vi "Motor_ReadPIDGains.vi"(8 "error in (no error)":errorcluster, 11 "MotorNew in":refnum<class "MotorControl.lvclass">) -> (0 "error out":errorcluster, 2 "PID Gains":T1(array[cluster]), 3 "MotorNew out":refnum<class "MotorControl.lvclass">)   [LabVIEW 2014, in "MotorControl.lvclass"]
uses:
  MotorControl.lvclass
  MotorControl.lvclass/MotorControl.ctl
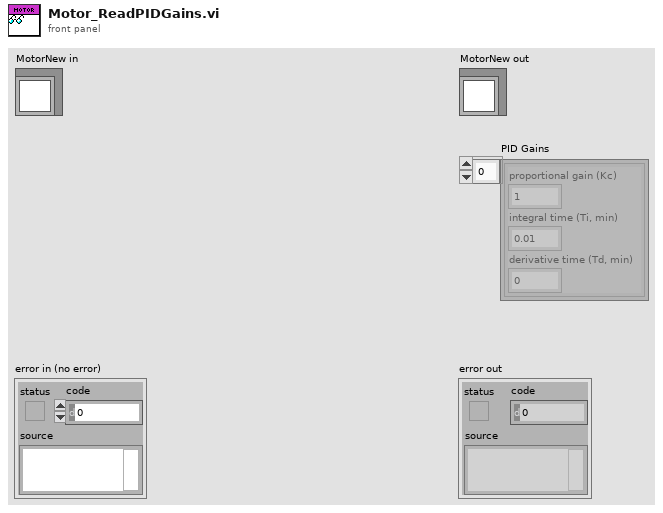
[diagram p1: front panel]
types:
  T1 = cluster{"proportional gain (Kc)":dbl, "integral time (Ti, min)":dbl, "derivative time (Td, min)":dbl}[]
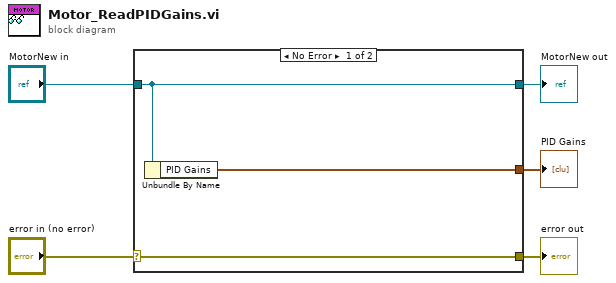
[diagram p0: block diagram]
diagram:
  n1 = case shown="No Error" "error in (no error)" {
    selector: "error in (no error)" -> [w8 w9]
    tunnel: [w8 w9] -> w4
    tunnel: [w7 w10] -> w2
    tunnel: "MotorNew in" -> [w7 w10]
    tunnel: [w6 _] -> w1
    frame No Error {
      n2 = Unbundle By Name(w7) -> ("PID Gains"=w6:T1)
    }
    frame Error {
    }
  }
  "error out" <- w4
  "MotorNew out" <- w2
  "PID Gains" <- w1
